vi "Voltage lvl indicator.vi"(9 "V3":dbl, 10 "V2":dbl, 11 "V1":dbl) -> (1 "?":u8(slide) scale=50.0..100.0, 2 "?":u8(slide) scale=50.0..100.0, 3 "?":u8(slide) scale=50.0..100.0)   [LabVIEW 2020]
doc: "Aesthetic purpose Vi - to fill bars"
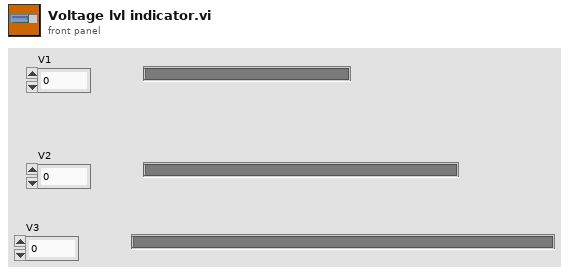
[diagram p1: front panel]
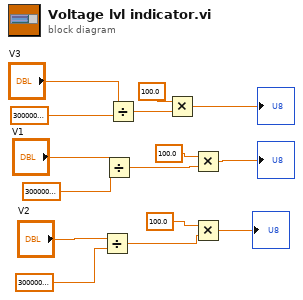
[diagram p0: block diagram]
diagram:
  n1 = Divide(x="V2", y=300000000000000.0) -> (x/y=w2:dbl)
  n2 = Divide(x="V1", y=300000000000000.0) -> (x/y=w4:dbl)
  n3 = Divide(x="V3", y=300000000000000.0) -> (x/y=w10:dbl)
  n4 = Multiply(x=100.0, y=w10) -> (x*y=→"?":dbl)
  n5 = Multiply(x=100.0, y=w4) -> (x*y=→"?":dbl)
  n6 = Multiply(x=100.0, y=w2) -> (x*y=→"?":dbl)
